vi "Speak.vi"(8 "Error In":errorcluster, 11 "reference in":refnum<class "Person.lvclass">) -> (0 "Error Out":errorcluster, 2 "Result":string, 3 "reference out":refnum<class "Person.lvclass">)   [LabVIEW 2024, in "Person.lvclass"]
uses:
  Person.lvclass
  Person.lvclass/Person.ctl
  ISpeakBehaviour/ISpeakBehaviour.lvclass
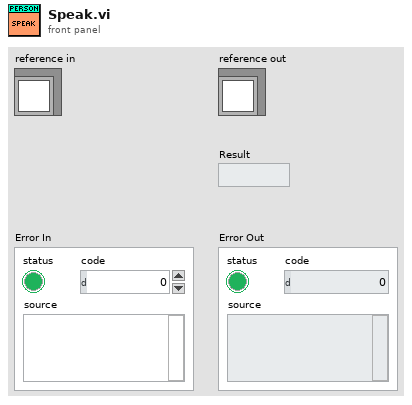
[diagram p1: front panel]
types:
  T1 = typedef "Person.lvclass/ObjectAttributes.ctl" = cluster{"SpeakBehaviour":refnum<class "ISpeakBehaviour.lvclass">, "LearnBehaviour":refnum<class "ILearnBehaviour.lvclass">, "Name":string}
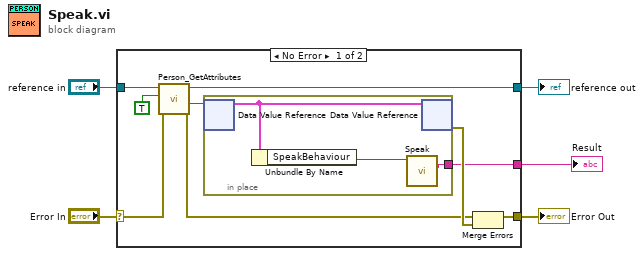
[diagram p0: block diagram]
diagram:
  n1 = case shown="No Error" "Error In" {
    selector: "Error In" -> [w13 w19]
    tunnel: [w10 w19] -> w4
    tunnel: [w11 w18] -> w2
    tunnel: "reference in" -> [w14 w18]
    tunnel: [w6 _] -> w1
    frame No Error {
      n2 = call "Person_GetAttributes.vi"("Error In"=w13, "OnlyGetDvrReference(False)"=TRUE, "reference in"=w14) -> ("Error Out"=w8:errorcluster, "DataRef"=w9:refnum<data-value>, "reference out"=w11:refnum<class "Person.lvclass">)  [unwired: 5 in, 1 out]
      n3 = in-place {
        in-place-border: [w15] -> w6
        n4 = in-place-dvr #1(w9) -> (w17:T1)  [unwired: 1 out]
        n5 = Unbundle By Name(w17) -> ("SpeakBehaviour"=w16:refnum<class "ISpeakBehaviour.lvclass">)
        n6 = call-dynamic "Speak.vi"("object in"=w16) -> ("Result"=w15:string)  [unwired: 8 in, 2 out]
        n7 = in-place-dvr #1(w17) -> (w12:errorcluster)  [unwired: 1 out]
      }
      n8 = Merge Errors(w8, w12) -> (w10:errorcluster)
    }
    frame Error {
    }
  }
  "Error Out" <- w4
  "reference out" <- w2
  "Result" <- w1
